vi "MRC Console Write Error.vi"(6 "stackTrace":T1, 7 "location":T1, 8 "error in (no error)":errorcluster, 9 "message":T1, 10 "errorCode":i32, 11 "isError":u8) -> (0 "error out":errorcluster)   [LabVIEW 2026, in "MrcLib.lvlib"]
doc: "MRC_Status MRC_CALLCONV MRC_Console_WriteError(\n MRC_Bool isError, int32_t errorCode, const struct MRC_String* message,\n const struct MRC_String* location, const struct MRC_String* stackTrace);"
uses:
  MrcLib.lvlib
  Types/MRC String.ctl
  MrcLib.dll
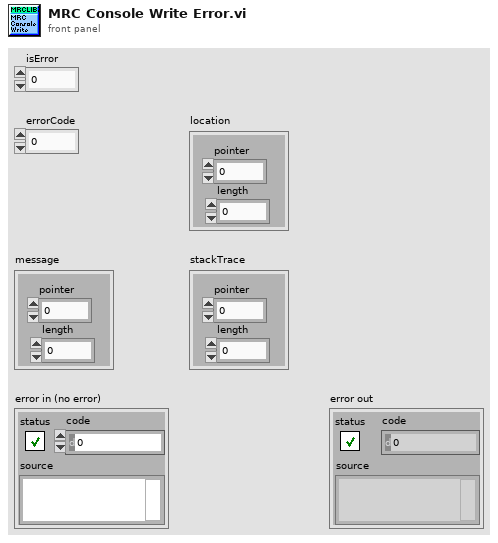
[diagram p1: front panel]
types:
  T1 = typedef "MRC String.ctl" = cluster{"pointer":u64, "length":u64}
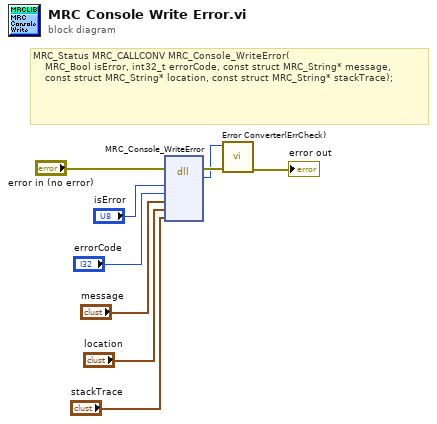
[diagram p0: block diagram]
diagram:
  # "MRC_Status MRC_CALLCONV MRC_Console_WriteError(\n    MRC_Bool isError, int32_t errorCode, const struct MRC_String* message,\n    const struct MRC_String* location, const struct MRC_String* stackTrace);"
  n1 = dll-call lib="MrcLib.*" fn="MRC_Console_WriteError"(error in="error in (no error)", "isError"="isError", "errorCode"="errorCode", "message"="message", "location"="location", "stackTrace"="stackTrace") -> (error out=w3:errorcluster, "return type"=w1:i32)  [unwired: 7 in, 1 out]
  n2 = call "Error Converter(ErrCheck).vi"("error in (no error)"=w3, "status"=w1) -> ("error out"=→"error out":errorcluster)  [unwired: 9 in]
